vi "Optimize 1D.vi"(5 "AO Channel":tag="Dev1/ao0", 7 "Fit Method":enum16{"Max", "Gaussian"}(ring), 8 "Dwell Time (ms)":i32=2, 9 "Volt Step":dbl, 10 "Volt Range":dbl, 11 "Curr Pos":dbl) -> (2 "Max Counts":dbl, 3 "Final Pos":dbl)   [LabVIEW 2012]
uses:
  <vilib>/Analysis/NI_AALPro.lvlib
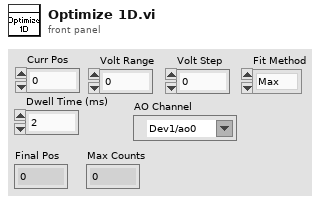
[diagram p1: front panel]
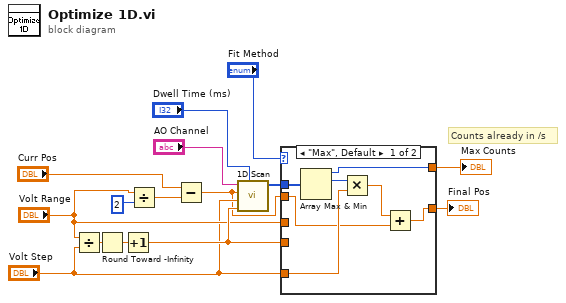
[diagram p0: block diagram]
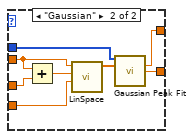
[diagram p2: hidden frame]
diagram:
  # "Counts already in /s"
  n1 = Divide(x="Volt Range", y="Volt Step") -> (x/y=w13:dbl)
  n2 = Round Toward -Infinity(1:w13) -> (0:w14:dbl)
  n3 = Increment(x=w14) -> (x+1=w8:dbl)
  n4 = Divide(x="Volt Range", y=2) -> (x/y=w12:dbl)
  n5 = Subtract(x="Curr Pos", y=w12) -> (x-y=w5:dbl)
  n6 = call "1D Scan.vi"("Dwell Time (ms)"="Dwell Time (ms)", "Num Steps"=w8, "Step"="Volt Step", "Min"=w5, "Channel"="AO Channel") -> ("Counts"=w10:i32[])  [unwired: 6 in]
  n7 = case shown="\"Max\", Default" "Fit Method" {
    tunnel: [w17 w30] -> w3
    tunnel: w10 -> [w21 w29]
    tunnel: "Volt Step" -> [w19 _]
    tunnel: w5 -> [w18 w26]
    tunnel: w8 -> [_ w27]
    tunnel: "Volt Range" -> [_ w25]
    tunnel: [w16 w23] -> w1
    frame "Max", Default {
      n8 = Array Max & Min(array=w21) -> (max value=w16:i32, max index (indices)=w20:i32)  [unwired: 2 out]
      n9 = Multiply(x=w20, y=w19) -> (x*y=w22:dbl)
      n10 = Add(x=w22, y=w18) -> (x+y=w17:dbl)
    }
    frame "Gaussian" {
      n11 = Add(x=w26, y=w25) -> (x+y=w24:dbl)
      n12 = call "LinSpace.vi"("Num Steps"=w27, "Max"=w24, "Min"=w26) -> ("Array"=w28:dbl[])  [unwired: 8 in]
      n13 = call <vilib>:"Gaussian Peak Fit.vi"("Y"=w29, "X"=w28) -> ("amplitude"=w23:dbl, "center"=w30:dbl)  [unwired: 7 in, 5 out]
    }
  }
  "Final Pos" <- w3
  "Max Counts" <- w1
